vi "Stop Core.vi"(10 "final error code":i32, 11 "Base Software in":refnum<class "Base Software.lvclass">) -> (3 "Base Software out":refnum<class "Base Software.lvclass">)   [LabVIEW 2019, in "Base Software.lvlib" / "Main.lvlib" / "Base Software.lvclass"]
doc: "This routine transmits a stop core message to all instantiated actors and calls the <b>Shutdown</b> routine."
uses:
  Project/Base Software.lvclass
  builds/Engine/Engine.lvlibp/Project/Engine.lvclass
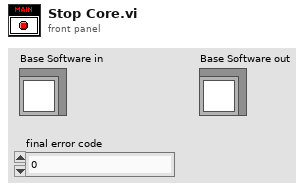
[diagram p1: front panel]
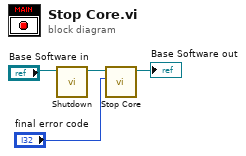
[diagram p0: block diagram]
diagram:
  n1 = call "Shutdown.vi"("Base Software in"="Base Software in") -> ("Base Software out"=w1:refnum<class "Base Software.lvclass">)  [unwired: 9 in, 1 out]
  n2 = call-parent "Stop Core.vi"("final error code"="final error code", "Monitored Actor in"=w1) -> ("Monitored Actor out"=→"Base Software out":refnum<class "Base Software.lvclass">)  [unwired: 9 in]
